vi "file -- get unique increment name.vi"(10 "prefix":string="image", 11 "9w folder path":path=path "C:/data/RUS/Experiment/ProbeTest/Probe10/YBCO_6/sweep2/9w") -> (1 "unique index out":i32)   [LabVIEW 2019]
uses:
  <vilib>/regexp/Match Regular Expression.xnode
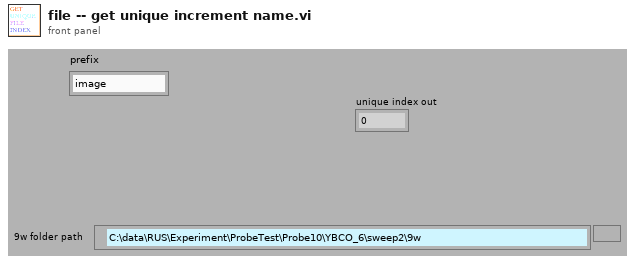
[diagram p1: front panel]
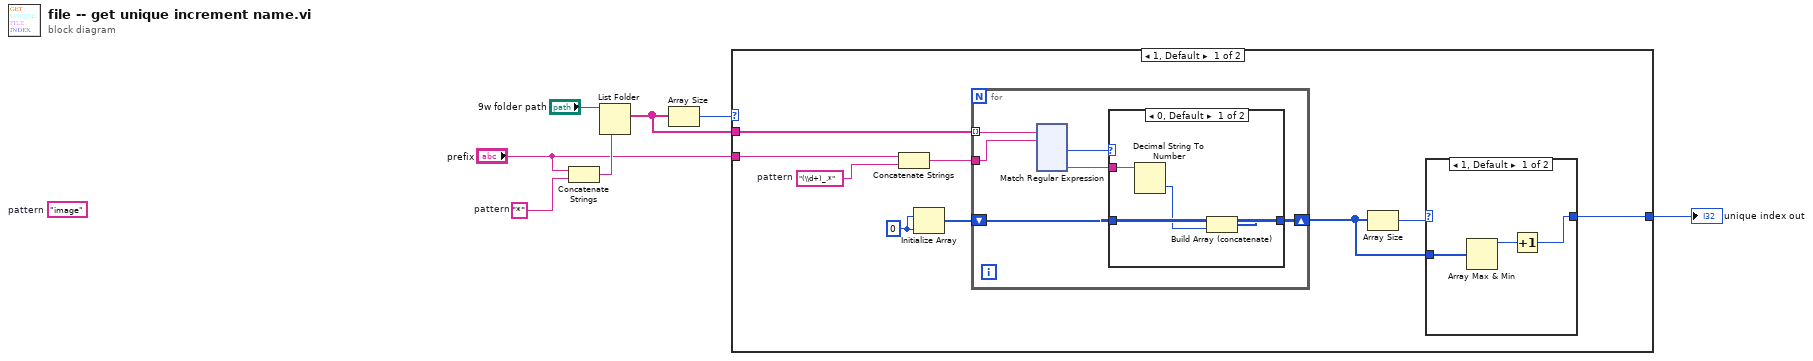
[diagram p0: block diagram]
diagram:
  w7 = "*"  # pattern
  (unwired) "image"  # pattern
  n1 = Concatenate Strings("prefix", w7) -> (w6:string)
  n2 = List Folder(path="9w folder path", pattern=w6) -> (filenames=w4:string[])  [unwired: 2 in, 3 out]
  n3 = Array Size(array=w4) -> (size(s)=w5:i32)
  n4 = case shown="1, Default" w5 {
    selector: w5 -> [_ w145]
    tunnel: "prefix" -> [w9 _]
    tunnel: w4 -> [w16 _]
    tunnel: [w11 w145] -> w3
    frame 1, Default {
      w13 = 0
      w8 = "(\\d+)_.*"  # pattern
      n5 = Concatenate Strings(w9, w8) -> (w15:string)
      n6 = Initialize Array(w13, w13) -> (w14:i32[])
      n7 = for {
        tunnel: w16 -> [w26] mode=indexing
        tunnel: w15 -> [w25]
        shift-right: [w23] -> w10
        shift-left: w14 -> [w22]
        n8 = xnode "Match Regular Expression"("input string"=w26, "regular expression"=w25) -> ("offset past match"=w24:i32, "submatch 1"=w21:string)  [unwired: 4 in, 4 out]
        n9 = case shown="0, Default" w24 {
          tunnel: [w29 w31] -> w23
          tunnel: w22 -> [w30 w31]
          tunnel: w21 -> [w28 _]
          frame 0, Default {
            n10 = Decimal String To Number(string=w28) -> (number=w27:i32)  [unwired: 2 in, 1 out]
            n11 = Build Array (concatenate)(w30, w27) -> (w29:i32[])
          }
          frame -1 {
          }
        }
      }
      n12 = Array Size(array=w10) -> (size(s)=w12:i32)
      n13 = case shown="1, Default" w12 {
        selector: w12 -> [_ w20]
        tunnel: [w17 w20] -> w11
        tunnel: w10 -> [w19 _]
        frame 1, Default {
          n14 = Array Max & Min(array=w19) -> (max value=w18:i32)  [unwired: 3 out]
          n15 = Increment(x=w18) -> (x+1=w17:i32)
        }
        frame 0 {
        }
      }
    }
    frame 0 {
    }
  }
  "unique index out" <- w3
